vi "Test Environment Chamber API.vi"() -> ()   [LabVIEW 2016]
doc: "Environment Chamber API Tester."
uses:
  Configure Parameter.ctl
  <vilib>/Utility/miscctls.llb/LVPointTypeDef.ctl
  <vilib>/Utility/error.llb/DialogType.ctl
  Environment Chamber.lvlib
panel:
  in  "REQ Retry EC":bool
  in  "REQ Wakeup_helper_loop":bool
  in  "REQ Close Ref":bool
  in  "REQ Acquire Humidity":bool
  in  "REQ Acquire Data":bool
  in  "Configure Parameter":T1={"Temp Parameter"={"Temperature setpoint"=40.0, "upper limit"=80.0, "lower limit"=0.0}, "Humidity Parameter"={"Humidity setpoint"=50.0, "upper limit"=80.0, "lower limit"=0.0}}
  in  "REQ Configure Parameter":bool
  in  "Connection Ref":refnum<visa-resource-name>
  out "Connect?":bool
  in  "REQ Initialize Hardware":bool
  in  "DAQ Type":enum16{"Hardware", "Simulation"}(ring)
  in  "Show Diagram on Init":bool
  in  "Show Block Diagram":bool
  in  "Stop Module":bool
  in  "Start Module":bool
  in  "Hide Module Panel":bool
  in  "Show Module Panel":bool
  out "Status":string
  out "Module Running?":bool
  # "This VI tests the API for the Module."
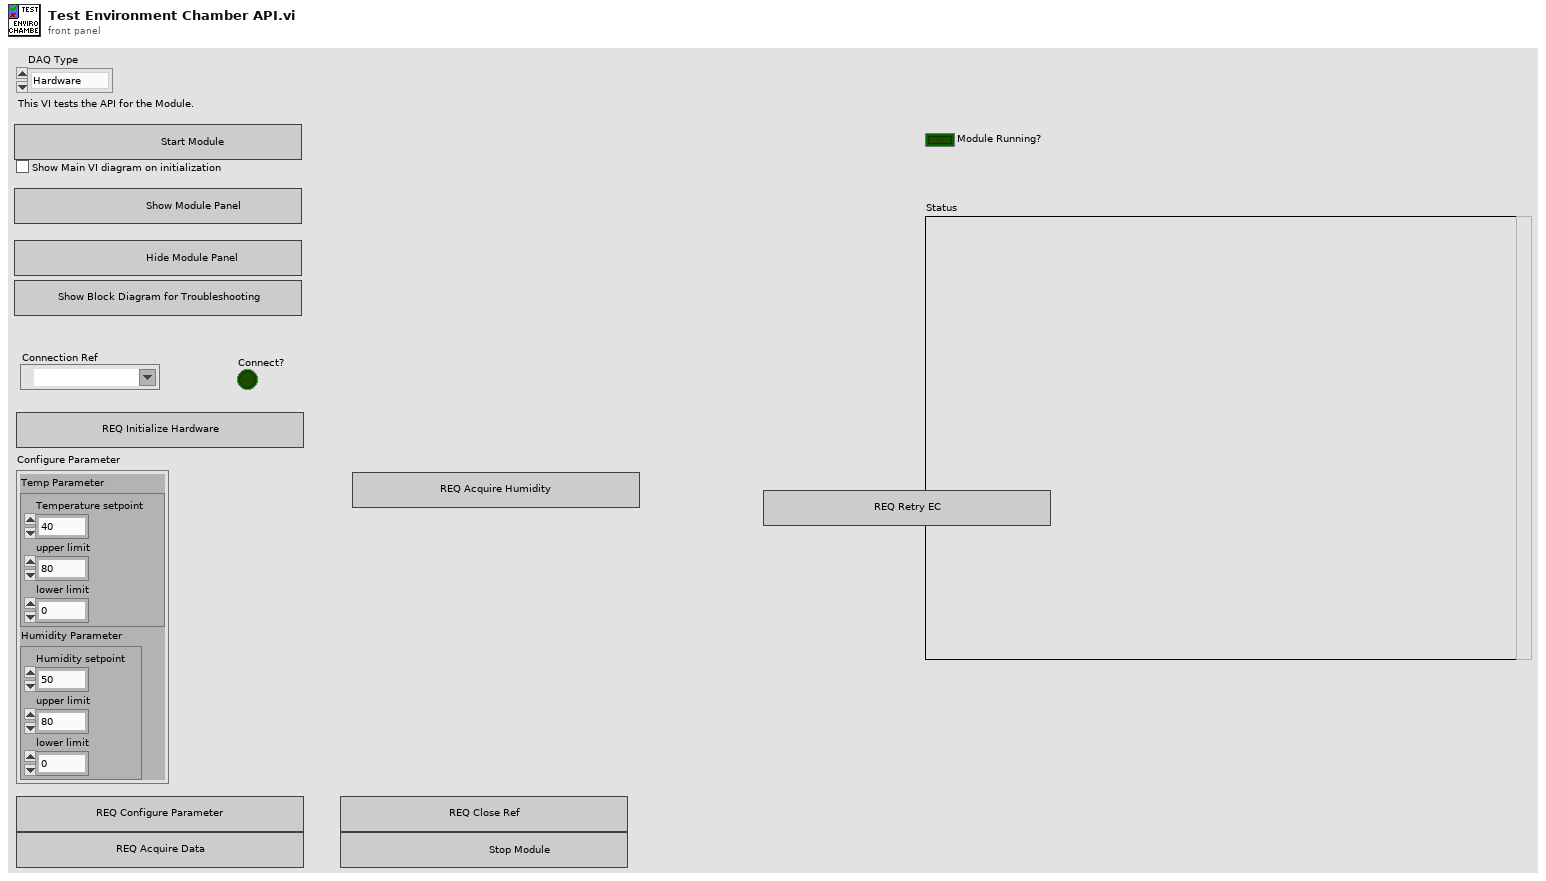
[diagram p1: front panel]
types:
  T1 = typedef "Environment Chamber.lvlib/Configure Parameter.ctl" = cluster{"Temp Parameter":cluster{"Temperature setpoint":dbl, "upper limit":dbl, "lower limit":dbl}, "Humidity Parameter":cluster{"Humidity setpoint":dbl, "upper limit":dbl, "lower limit":dbl}}
  T2 = typedef "LVPointTypeDef.ctl" = cluster{"Horizontal":i16, "Vertical":i16}
  T3 = typedef "Environment Chamber.lvlib/Broadcast Events--cluster.ctl" = cluster{"Module Did Init":refnum<user-event>, "Status Updated":refnum<user-event>, "Error Reported":refnum<user-event>, "Module Did Stop":refnum<user-event>, "Update Module Execution Status":refnum<user-event>, "Broad Temp Data":refnum<user-event>, "Broad Humidity. Data":refnum<user-event>}
  T4 = typedef "DialogType.ctl" = u16
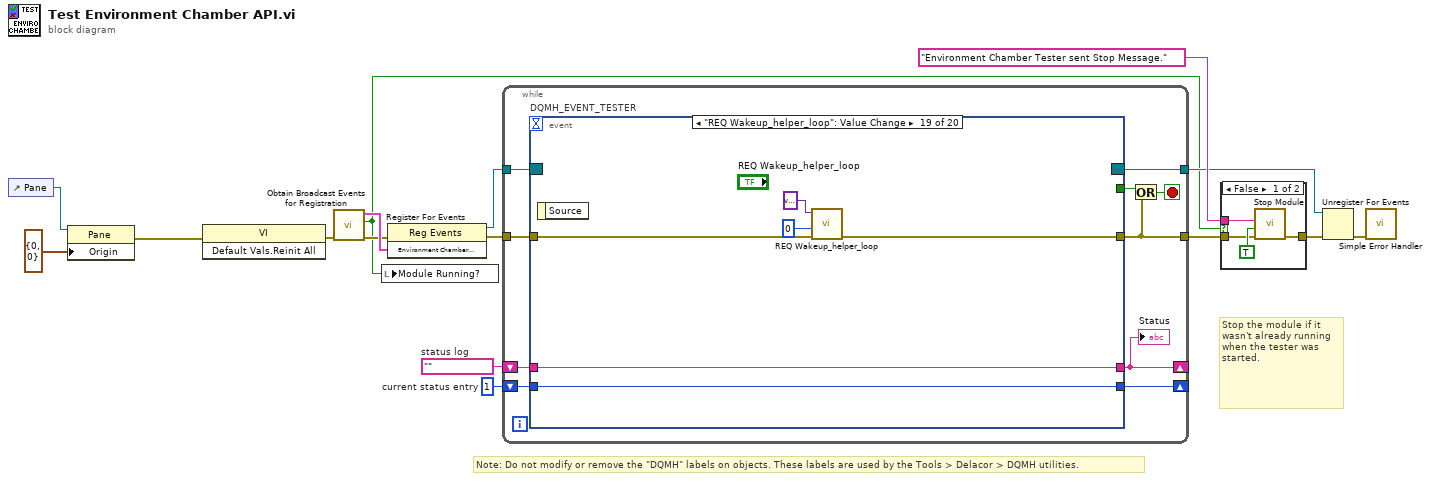
[diagram p0: block diagram]
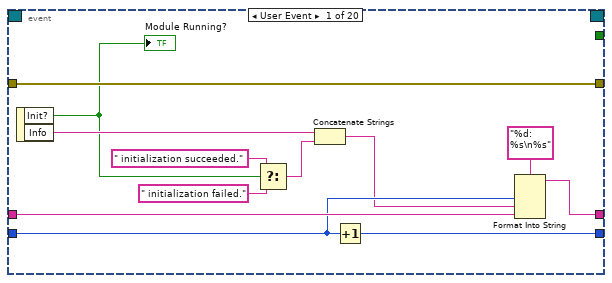
[diagram p3: hidden frame]
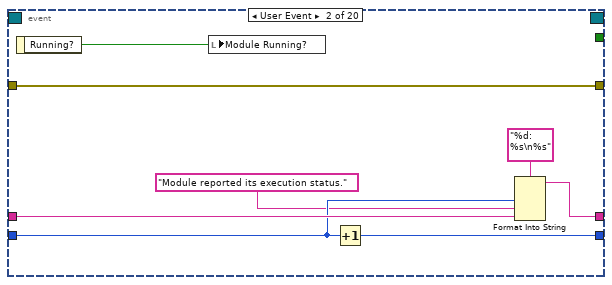
[diagram p4: hidden frame]
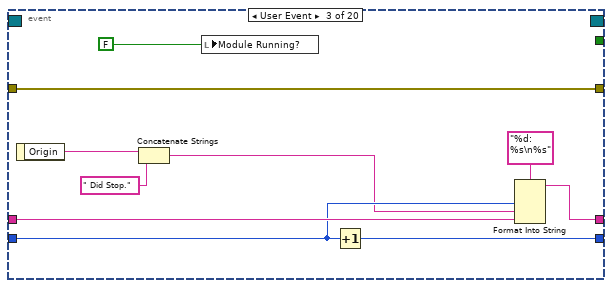
[diagram p5: hidden frame]
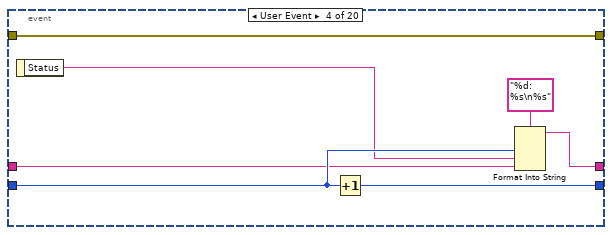
[diagram p6: hidden frame]
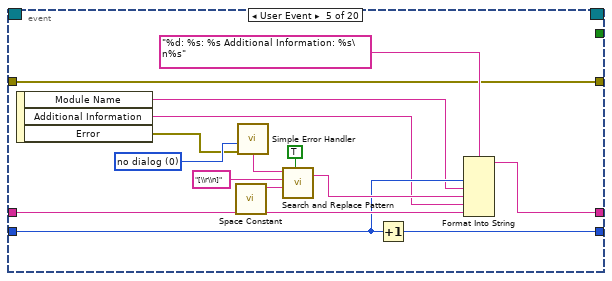
[diagram p7: hidden frame]
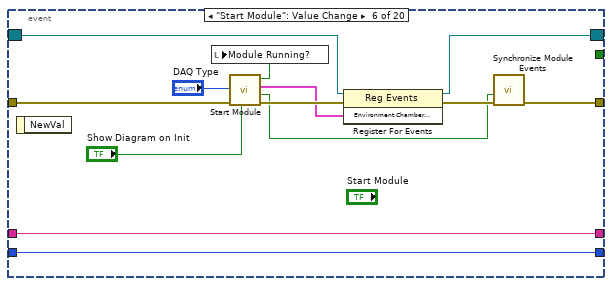
[diagram p8: hidden frame]
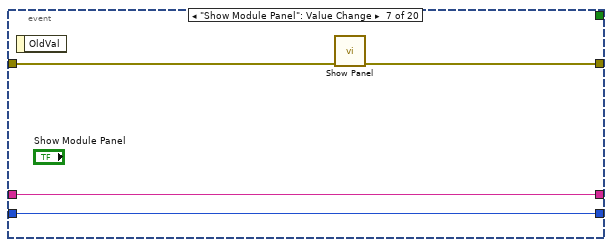
[diagram p9: hidden frame]
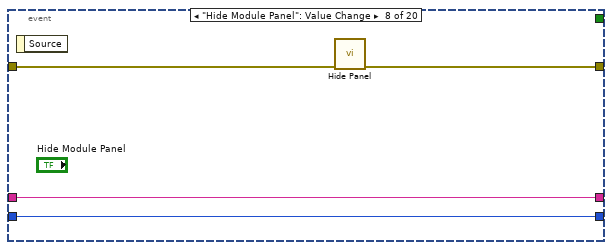
[diagram p10: hidden frame]
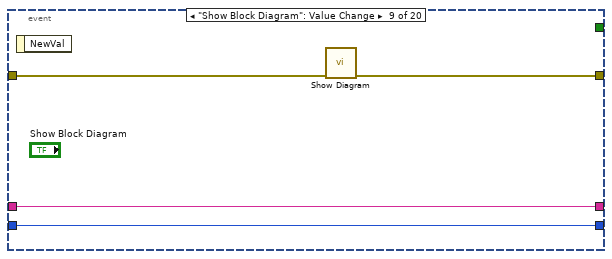
[diagram p11: hidden frame]
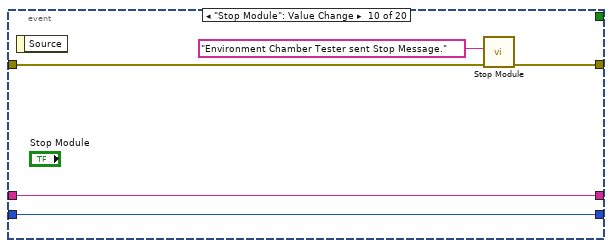
[diagram p12: hidden frame]
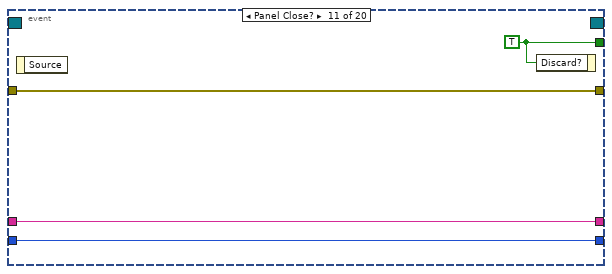
[diagram p13: hidden frame]
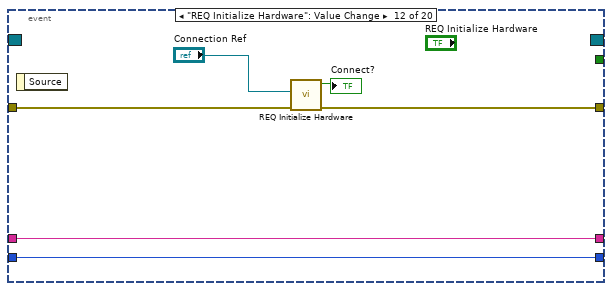
[diagram p14: hidden frame]
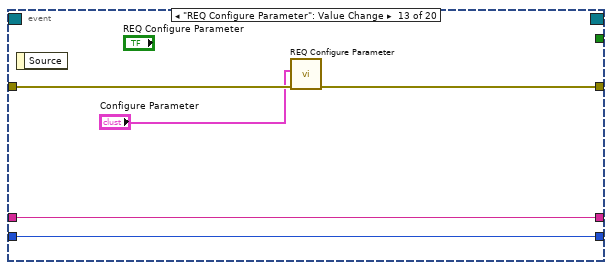
[diagram p15: hidden frame]
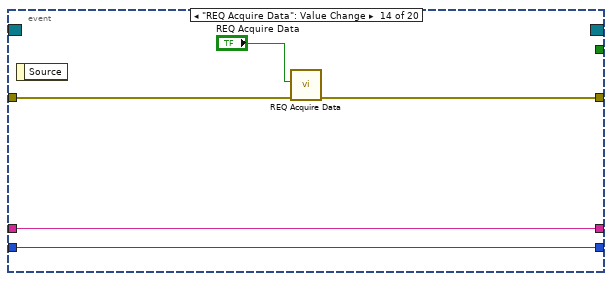
[diagram p16: hidden frame]
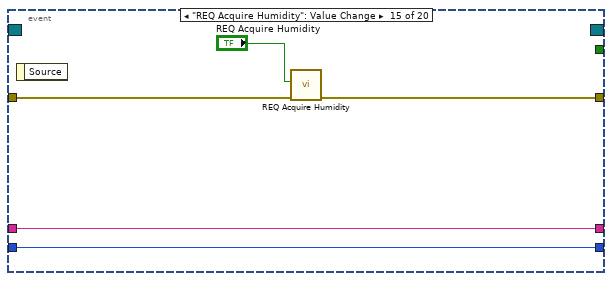
[diagram p17: hidden frame]
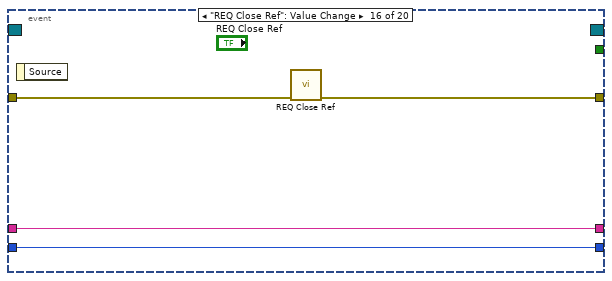
[diagram p18: hidden frame]
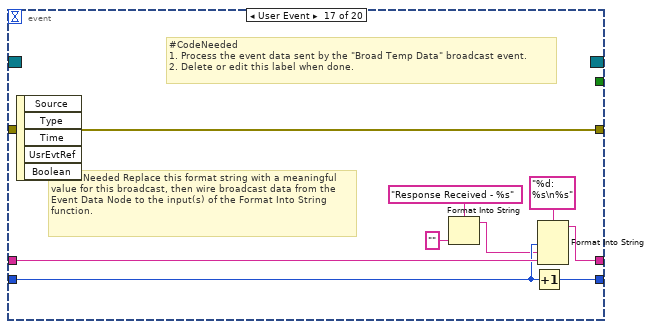
[diagram p19: hidden frame]
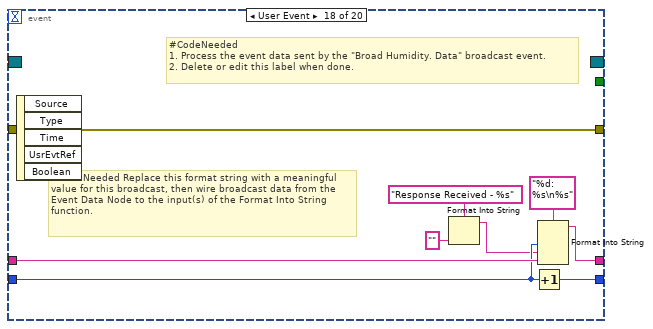
[diagram p20: hidden frame]
diagram:
  w13 = 1  # current status entry
  w14 = ""  # status log
  # "Stop the module if it wasn't already running when the tester was started."
  # "Note: Do not modify or remove the \"DQMH\" labels on objects. These labels are used by the Tools > Delacor > DQMH utilities."
  n1 = control-ref of="Pane"() -> (w2:refnum<vi>)
  n2 = property class="Pane"(reference=w2, "Origin"=T2 {"Horizontal"=0, "Vertical"=0}) -> (error out=w3:errorcluster)  [unwired: 1 in, 1 out]
  n3 = invoke class="VI" method="Default Vals.Reinit All"(error in=w3) -> (error out=w8:errorcluster)  [unwired: 2 in, 2 out]
  n4 = call "Obtain Broadcast Events for Registration.vi"("error in"=w8) -> ("error out"=w7:errorcluster, "Already running?"=w6:bool, "Environment Chamber Broadcast Events"=w11:T3)  [unwired: 8 in]
  n5 = local write "Module Running?"(w6) -> ()
  n6 = register-events(error in=w7, w11) -> (reference out=w10:refnum<event-registration>, error out=w12:errorcluster)  [unwired: 1 in]
  n7 = while {
    tunnel: w10 -> [w26]
    tunnel: [w17] -> w5
    shift-right: [w21] -> _
    shift-left: w14 -> [w23]
    shift-right: [w22] -> _
    shift-left: w13 -> [w24]
    tunnel: w12 -> [w19]
    tunnel: [w18] -> w9
    stop <- w20 stop-if-true
    n8 = event "DQMH_EVENT_TESTER" shown="[18] \"REQ Wakeup_helper_loop\": Value Change" {
      selector: w26 -> [_ _ _ _ _ w85 _ _ _ _ _ _ _ _ _ _ _ _ _ _]
      dyn-events: [_ _ _ _ _ w84 _ _ _ _ _ _ _ _ _ _ _ _ _ _] -> w18
      timeout: _ -> [_ _ _ _ _ _ _ _ _ _ _ _ _ _ _ _ _ _ _ _]
      tunnel: [_ _ _ _ _ _ _ _ _ _ w112 _ _ _ _ _ _ _ _ _] -> w25
      tunnel: [w38 w40 w47 w57 w67 w83 w95 w99 w100 w106 w109 w115 w120 w125 w130 w134 w146 w155 w158 w162] -> w17
      tunnel: w24 -> [w35 w44 w54 w60 w70 w88 w93 w97 w101 w107 w110 w116 w121 w126 w131 w135 w143 w152 w159 w163]
      tunnel: w23 -> [w36 w45 w55 w59 w71 w89 w94 w98 w102 w108 w111 w117 w122 w127 w132 w136 w145 w154 w160 w164]
      tunnel: [w33 w42 w52 w61 w69 w89 w94 w98 w102 w108 w111 w117 w122 w127 w132 w136 w144 w153 w160 w164] -> w21
      tunnel: [w34 w43 w53 w63 w68 w88 w93 w97 w101 w107 w110 w116 w121 w126 w131 w135 w142 w151 w159 w163] -> w22
      tunnel: w19 -> [w38 w40 w47 w57 w67 w82 w92 w96 w103 w104 w109 w118 w123 w128 w133 w137 w146 w155 w161 w165]
      event User Event {
        n9 = event-data() -> ("Init?"=w30:bool, "Info"=w32:string)  [unwired: 1 in]
        "Module Running?" <- w30
        n10 = Select(t=" initialization succeeded.", s=w30, f=" initialization failed.") -> (s? t:f=w27:string)
        n11 = Concatenate Strings(w32, w27) -> (w31:string)
        n12 = Increment(x=w35) -> (x+1=w34:i32)
        n13 = Format Into String(format string="%d: %s\n%s", w35, w31, w36) -> (resulting string=w33:string)  [unwired: 2 in, 1 out]
      }
      event User Event {
        n14 = event-data() -> ("Running?"=w39:bool)  [unwired: 1 in]
        n15 = local write "Module Running?"(w39) -> ()
        n16 = Increment(x=w44) -> (x+1=w43:i32)
        n17 = Format Into String(format string="%d: %s\n%s", w44, "Module reported its execution status.", w45) -> (resulting string=w42:string)  [unwired: 2 in, 1 out]
      }
      event User Event {
        n18 = event-data() -> ("Origin"=w51:string)  [unwired: 1 in]
        n19 = Concatenate Strings(w51, " Did Stop.") -> (w50:string)
        n20 = local write "Module Running?"(FALSE ("Module Did Init?")) -> ()
        n21 = Increment(x=w54) -> (x+1=w53:i32)
        n22 = Format Into String(format string="%d: %s\n%s", w54, w50, w55) -> (resulting string=w52:string)  [unwired: 2 in, 1 out]
      }
      event User Event {
        n23 = event-data() -> ("Status"=w58:string)  [unwired: 1 in]
        n24 = Increment(x=w60) -> (x+1=w63:i32)
        n25 = Format Into String(format string="%d: %s\n%s", w60, w58, w59) -> (resulting string=w61:string)  [unwired: 2 in, 1 out]
      }
      event User Event {
        w72 = T4 0 items=["no dialog", "OK message", "continue or stop message", "OK message + warnings", "continue/stop + warnings"] ("type of dialog (OK msg:1)")
        n26 = event-data() -> ("Module Name"=w66:string, "Additional Information"=w65:string, "Error"=w64:errorcluster)  [unwired: 1 in]
        n27 = call <vilib>:"Space Constant.vi"() -> ("String"=w76:string)
        n28 = call <vilib>:"Simple Error Handler.vi"("type of dialog (OK msg:1)"=w72, "error in (no error)"=w64) -> ("message"=w73:string)  [unwired: 3 in, 4 out]
        n29 = call <vilib>:"Search and Replace Pattern.vi"("string"=w73, "regular expression (\"\")"="[\\r\\n]" ("regular expression (\"\")"), "replace string (\"\")"=w76, "replace all? (F)"=TRUE ("replace all CR/LF with spaces")) -> ("result string"=w74:string)  [unwired: 1 in, 1 out]
        n30 = Increment(x=w70) -> (x+1=w68:i32)
        n31 = Format Into String(format string="%d: %s: %s Additional Information: %s\n%s", w70, w66, w74, w65, w71) -> (resulting string=w69:string)  [unwired: 2 in, 1 out]
      }
      event "Start Module": Value Change {
        n32 = event-data() -> ()  [unwired: 1 in, 1 out]
        n33 = call "Start Module.vi"("Show Main VI Diagram on Init (F)"="Show Diagram on Init", "error in"=w82, "DAQ Type"="DAQ Type") -> ("error out"=w90:errorcluster, "Wait for Event Sync?"=w87:bool, "Environment Chamber Broadcast Events"=w86:T3, "Module Was Already Running?"=w81:bool)  [unwired: 5 in]
        n34 = local write "Module Running?"(w81) -> ()
        n35 = register-events(reference=w85, error in=w90, w86) -> (reference out=w84:refnum<event-registration>, error out=w91:errorcluster)
        n36 = call "Synchronize Module Events.vi"("error in"=w91, "Wait for Event Sync?"=w87) -> ("error out"=w83:errorcluster)  [unwired: 9 in]
      }
      event "Show Module Panel": Value Change {
        n37 = event-data() -> ()  [unwired: 1 in, 1 out]
        n38 = call "Show Panel.vi"("error in (no error)"=w92) -> ("error out"=w95:errorcluster)  [unwired: 10 in]
      }
      event "Hide Module Panel": Value Change {
        n39 = event-data() -> ()  [unwired: 1 in, 1 out]
        n40 = call "Hide Panel.vi"("error in (no error)"=w96) -> ("error out"=w99:errorcluster)  [unwired: 10 in]
      }
      event "Show Block Diagram": Value Change {
        n41 = event-data() -> ()  [unwired: 1 in, 1 out]
        n42 = call "Show Diagram.vi"("error in (no error)"=w103) -> ("error out"=w100:errorcluster)  [unwired: 10 in]
      }
      event "Stop Module": Value Change {
        n43 = event-data() -> ()  [unwired: 1 in, 1 out]
        n44 = call "Stop Module.vi"("error in"=w104, "Origin"="Environment Chamber Tester sent Stop Message.") -> ("error out"=w106:errorcluster)  [unwired: 9 in]
      }
      event Panel Close? {
        w112 = TRUE ("Discard?")
        n45 = event-data() -> ()  [unwired: 1 in, 1 out]
        n46 = event-data("Discard?"=w112) -> ()  [unwired: 1 in, 1 out]
      }
      event "REQ Initialize Hardware": Value Change {
        n47 = event-data() -> ()  [unwired: 1 in, 1 out]
        n48 = call "REQ Initialize Hardware.vi"("error in"=w118, "Connection Ref"="Connection Ref") -> ("error out"=w115:errorcluster, "Connect?"=→"Connect?":bool)  [unwired: 7 in, 1 out]
      }
      event "REQ Configure Parameter": Value Change {
        n49 = event-data() -> ()  [unwired: 1 in, 1 out]
        n50 = call "REQ Configure Parameter.vi"("error in"=w123, "Configure Parameter"="Configure Parameter") -> ("error out"=w120:errorcluster)  [unwired: 9 in]
      }
      event "REQ Acquire Data": Value Change {
        n51 = event-data() -> ()  [unwired: 1 in, 1 out]
        n52 = call "REQ Acquire Data.vi"("error in"=w128, "Acquire Data"="REQ Acquire Data") -> ("error out"=w125:errorcluster)  [unwired: 9 in]
      }
      event "REQ Acquire Humidity": Value Change {
        n53 = event-data() -> ()  [unwired: 1 in, 1 out]
        n54 = call "REQ Acquire Humidity.vi"("error in"=w133, "Acquire Humidity"="REQ Acquire Humidity") -> ("error out"=w130:errorcluster)  [unwired: 9 in]
      }
      event "REQ Close Ref": Value Change {
        n55 = event-data() -> ()  [unwired: 1 in, 1 out]
        n56 = call "REQ Close Ref.vi"("error in"=w137) -> ("error out"=w134:errorcluster)  [unwired: 10 in]
      }
      event User Event {
        # "#CodeNeeded Replace this format string with a meaningful value for this broadcast, then wire broadcast data from the Event Data Node to the input(s) of the Format Into String function."
        # "#CodeNeeded\n1. Process the event data sent by the \"Broad Temp Data\" broadcast event.\n2. Delete or edit this label when done."
        n57 = event-data() -> ()  [unwired: 1 in, 5 out]
        n58 = Format Into String(format string="Response Received - %s", "" ("input 1")) -> (resulting string=w139:string)  [unwired: 2 in, 1 out]
        n59 = Increment(x=w143) -> (x+1=w142:i32)
        n60 = Format Into String(format string="%d: %s\n%s", w143, w139, w145) -> (resulting string=w144:string)  [unwired: 2 in, 1 out]
      }
      event User Event {
        # "#CodeNeeded Replace this format string with a meaningful value for this broadcast, then wire broadcast data from the Event Data Node to the input(s) of the Format Into String function."
        # "#CodeNeeded\n1. Process the event data sent by the \"Broad Humidity. Data\" broadcast event.\n2. Delete or edit this label when done."
        n61 = event-data() -> ()  [unwired: 1 in, 5 out]
        n62 = Format Into String(format string="Response Received - %s", "" ("input 1")) -> (resulting string=w148:string)  [unwired: 2 in, 1 out]
        n63 = Increment(x=w152) -> (x+1=w151:i32)
        n64 = Format Into String(format string="%d: %s\n%s", w152, w148, w154) -> (resulting string=w153:string)  [unwired: 2 in, 1 out]
      }
      event "REQ Wakeup_helper_loop": Value Change {
        n65 = event-data() -> ()  [unwired: 1 in, 1 out]
        n66 = call "REQ Wakeup_helper_loop.vi"("error in"=w161, "Timeout"=0, "Data"=variant) -> ("error out"=w158:errorcluster)  [unwired: 8 in]
      }
      event "REQ Retry EC": Value Change {
        n67 = event-data() -> ()  [unwired: 1 in, 1 out]
        n68 = call "REQ Retry EC.vi"("error in"=w165) -> ("error out"=w162:errorcluster)  [unwired: 10 in]
      }
    }
    "Status" <- w21
    n69 = Or(x=w25, y=w17) -> (x .or. y?=w20:bool)
  }
  n70 = case shown="False" w6 {
    tunnel: [w169 w170] -> w16
    tunnel: "Environment Chamber Tester sent Stop Message." ("Origin") -> [w168 _]
    tunnel: w5 -> [w166 w170]
    frame False {
      n71 = call "Stop Module.vi"("error in"=w166, "Wait for Module to Stop? (F)"=TRUE ("Wait for Module to stop?"), "Origin"=w168) -> ("error out"=w169:errorcluster)  [unwired: 8 in]
    }
    frame True {
    }
  }
  n72 = Unregister For Events(event registration refnum=w9, error in=w16) -> (error out=w4:errorcluster)
  n73 = call <vilib>:"Simple Error Handler.vi"("error in (no error)"=w4) -> ()  [unwired: 4 in, 5 out]
